vi "Player Hand History Analyzer.vi"() -> ()   [LabVIEW 2020]
panel:
  out "Card Map":T1(array[cluster]) {"Average Profit/Loss (BBs)" format="%#_3g"}
  out "Overall Profit/Loss (BBs)":dbl
  out "Total Hands":i32
  out "Shown Hands":string[](array[string])
  in  "Player":string
  # "SUITED"
  # "OFFSUIT"
  # "A"
  # "K"
  # "Q"
  # "J"
  # "T"
  # "9"
  # "8"
  # "7"
  # "6"
  # "5"
  # "4"
  # "3"
  # "2"
  # "2"
  # "3"
  # "4"
  # "5"
  # "6"
  # "7"
  # "8"
  # "9"
  # "T"
  # "J"
  # "Q"
  # "K"
  # "A"
  # "A"
  # "K"
  # "Q"
  # "J"
  # "T"
  # "9"
  # "8"
  # "7"
  # "6"
  # "5"
  # "4"
  # "3"
  # "2"
  # "2"
  # "3"
  # "4"
  # "5"
  # "6"
  # "7"
  # "8"
  # "9"
  # "T"
  # "J"
  # "Q"
  # "K"
  # "A"
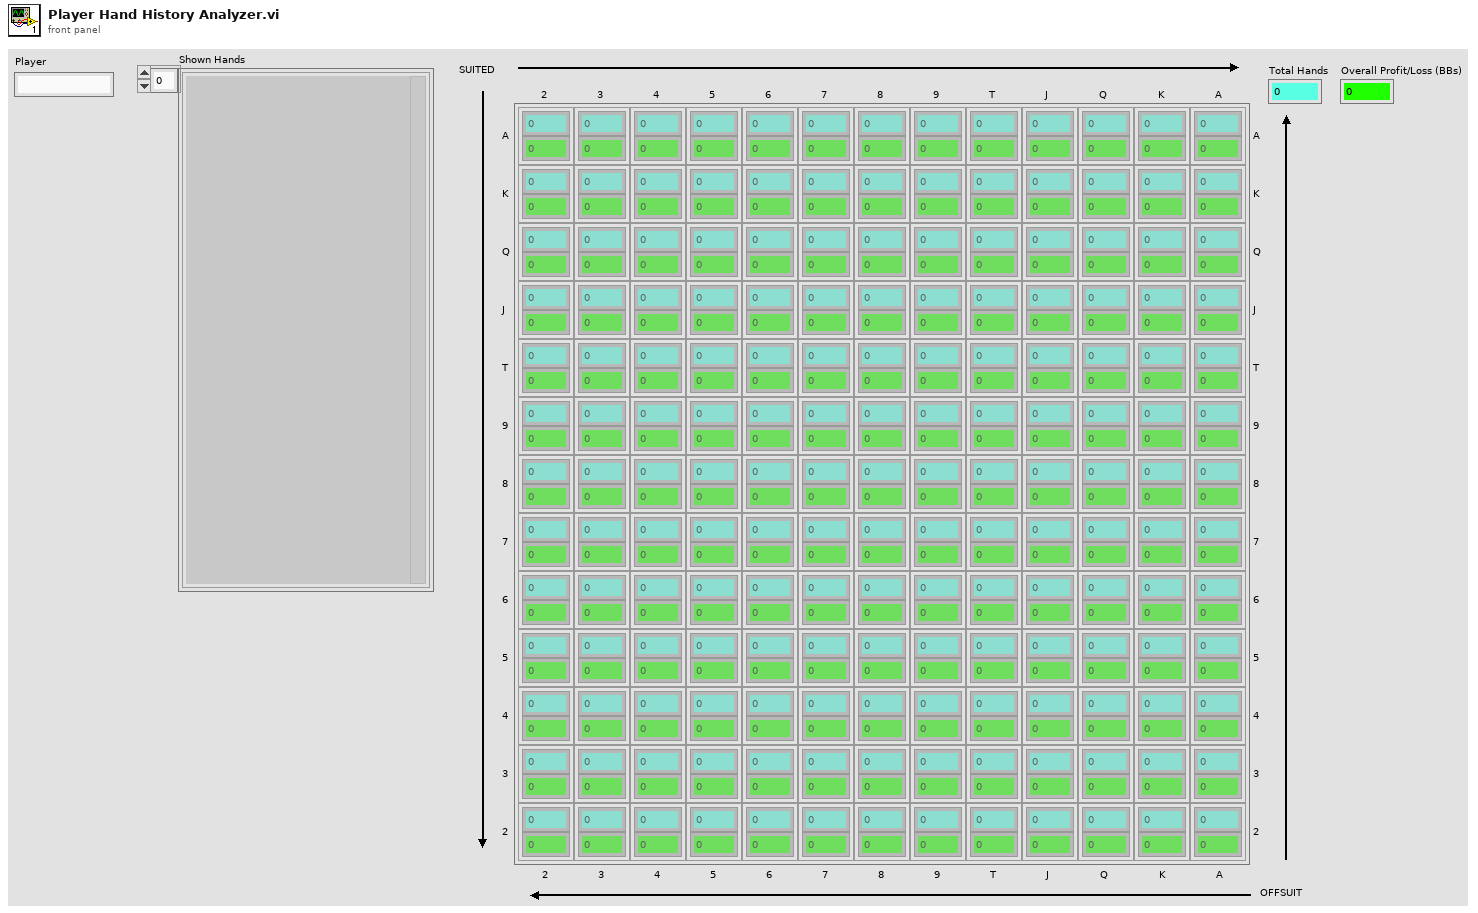
[diagram p1: front panel]
types:
  T1 = cluster{"Hand Count":u16, "Average Profit/Loss (BBs)":dbl}[][]
  T2 = cluster{"Hand Count":u16, "Average Profit/Loss (BBs)":dbl}
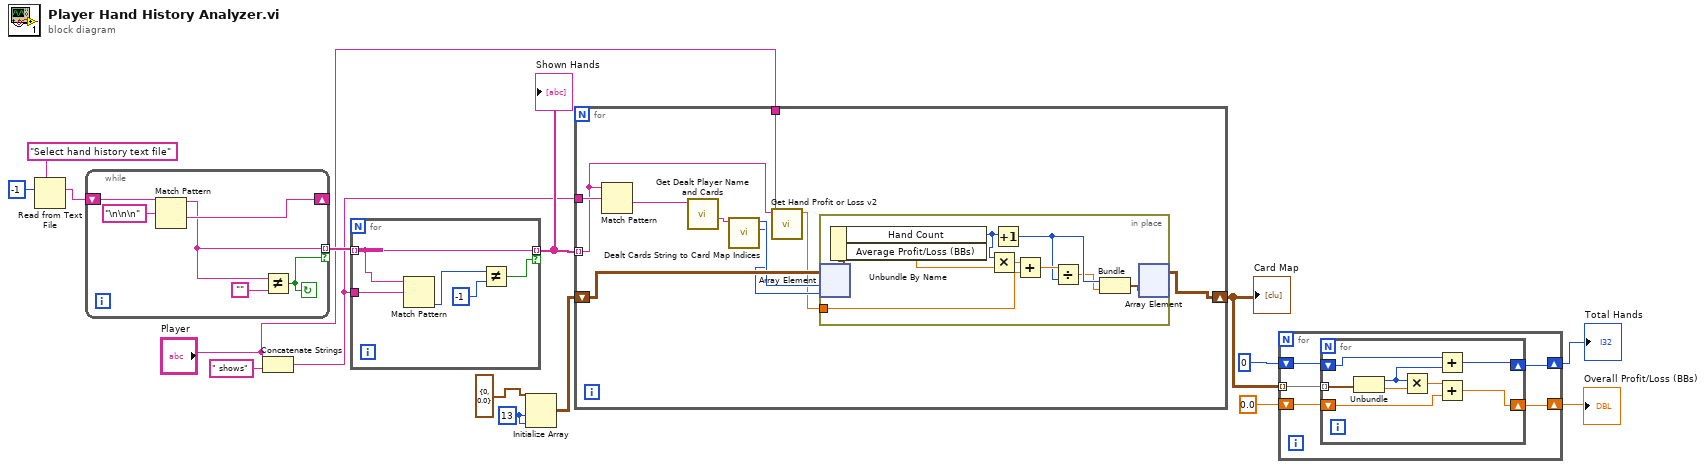
[diagram p0: block diagram]
diagram:
  w10 = 13 ("dimension size")
  n1 = Read from Text File(prompt (Open existing file)="Select hand history text file", count=-1) -> (text=w14:string)  [unwired: 2 in, 3 out]
  n2 = while {
    shift-right: [w21] -> _
    shift-left: w14 -> [w22]
    tunnel: [w19] -> w12 mode=indexing if=w17
    stop <- w17 continue-if-true
    n3 = Match Pattern(string=w22, regular expression="\n\n\n") -> (before substring=w19:string, after substring=w21:string)  [unwired: 1 in, 2 out]
    n4 = Not Equal?(x=w19, y="") -> (x != y?=w17:bool)
  }
  n5 = Concatenate Strings("Player", " shows" ("string")) -> (w7:string)
  n6 = for {
    tunnel: w12 -> [w23] mode=indexing
    tunnel: w7 -> [w27]
    tunnel: [w23] -> w11 mode=indexing if=w26
    n7 = Match Pattern(string=w23, regular expression=w27) -> (offset past match=w25:i32)  [unwired: 1 in, 3 out]
    n8 = Not Equal?(x=w25, y=-1) -> (x != y?=w26:bool)
  }
  "Shown Hands" <- w11
  n9 = Initialize Array(T2 {"Hand Count"=0, "Average Profit/Loss (BBs)"=0.0} ("Cluster"), w10, w10) -> (w8:T1)
  n10 = for {
    tunnel: w11 -> [w35] mode=indexing
    shift-right: [w32] -> w3
    shift-left: w8 -> [w33]
    tunnel: w7 -> [w36]
    tunnel: "Player" -> [w34]
    n11 = Match Pattern(string=w35, regular expression=w36) -> (after substring=w37:string)  [unwired: 1 in, 3 out]
    n12 = call "Get Dealt Player Name and Cards.vi"("Hand History String in"=w37) -> ("Dealt Cards"=w31:string)  [unwired: 8 in, 2 out]
    n13 = call "Dealt Cards String to Card Map Indices.vi"("Dealt Cards String"=w31) -> ("Index1"=w29:i32, "Index0"=w30:i32)  [unwired: 9 in]
    n14 = call "Get Hand Profit or Loss v2.vi"("Dealt Player Name"=w34, "Hand History String"=w35) -> ("Profit/Loss (BBs)"=w28:dbl)  [unwired: 9 in]
    n15 = in-place {
      in-place-border: w28 -> [w45]
      n16 = in-place-array #1(w33, w30, w29) -> (w38:T2)
      n17 = Unbundle By Name(w38) -> ("Hand Count"=w40:u16, "Average Profit/Loss (BBs)"=w41:dbl)
      n18 = Multiply(x=w40, y=w41) -> (x*y=w46:dbl)
      n19 = Increment(x=w40) -> (x+1=w43:u16)
      n20 = Add(x=w46, y=w45) -> (x+y=w44:dbl)
      n21 = Divide(x=w44, y=w43) -> (x/y=w42:dbl)
      n22 = Bundle(w43, w42) -> (w39:cluster{u16, dbl})  [unwired: 1 in]
      n23 = in-place-array #1(w39) -> (w32:T1)  [unwired: 2 out]
    }
  }
  "Card Map" <- w3
  n24 = for {
    tunnel: w3 -> [w51] mode=indexing
    shift-right: [w49] -> w2
    shift-left: 0.0 -> [w50]
    shift-right: [w47] -> w1
    shift-left: 0 -> [w48]
    n25 = for {
      tunnel: w51 -> [w59] mode=indexing
      shift-right: [w55] -> w49
      shift-left: w50 -> [w56]
      shift-right: [w52] -> w47
      shift-left: w48 -> [w54]
      n26 = Unbundle(w59) -> ("Hand Count"=w53:u16, "Average Profit/Loss (BBs)"=w58:dbl)
      n27 = Multiply(x=w53, y=w58) -> (x*y=w57:dbl)
      n28 = Add(x=w54, y=w53) -> (x+y=w52:i32)
      n29 = Add(x=w57, y=w56) -> (x+y=w55:dbl)
    }
  }
  "Total Hands" <- w1
  "Overall Profit/Loss (BBs)" <- w2
